vi "CountTeeth.vi"(8 "Falling Threshold":dbl, 9 "Rising Threshold":dbl, 10 "Direction":bool, 11 "Array":dbl[](array[numeric])) -> (0 "Gear Count":i32)   [LabVIEW 2017]
uses:
  ToothState.ctl
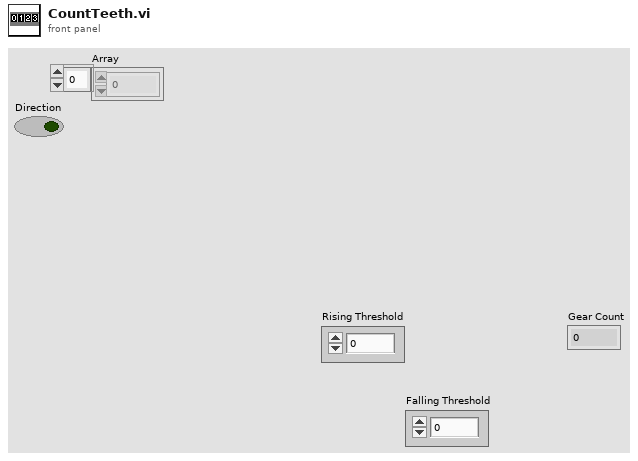
[diagram p1: front panel]
types:
  T1 = typedef "ToothState.ctl" = enum16{"Initialize State", "Rising ", "Falling"}
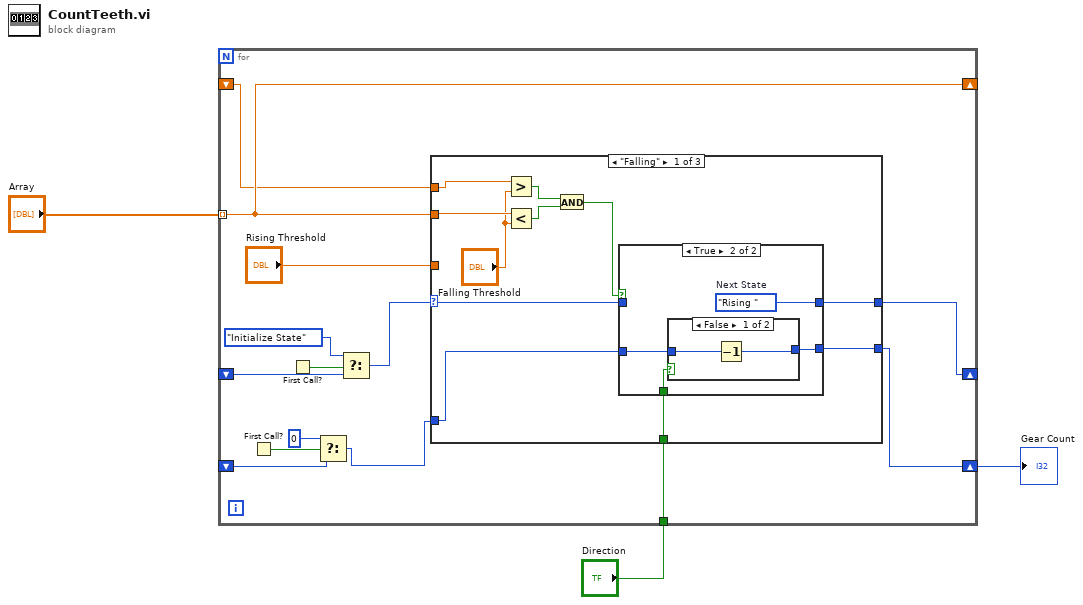
[diagram p0: block diagram]
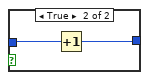
[diagram p3: hidden frame]
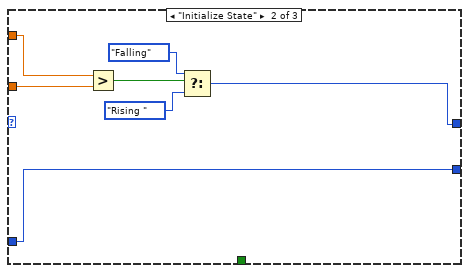
[diagram p4: hidden frame]
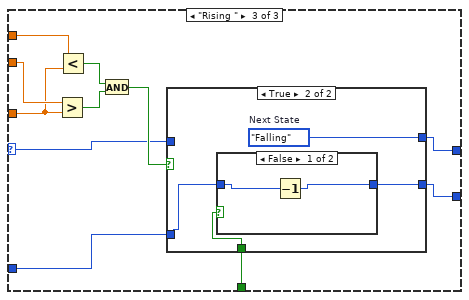
[diagram p5: hidden frame]
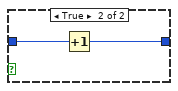
[diagram p7: hidden frame]
diagram:
  n1 = for {
    tunnel: "Array" -> [w17] mode=indexing
    shift-right: [w17] -> _
    shift-left: _ -> [w16]
    shift-right: [w15] -> _
    shift-left: _ -> [w11]
    shift-right: [w6] -> w3
    shift-left: _ -> [w7]
    tunnel: "Direction" -> [w5]
    n2 = First Call?() -> (First Call?: T/F=w9:bool)
    n3 = First Call?() -> (First Call?: T/F=w13:bool)
    n4 = Select(t=0, s=w9, f=w7) -> (s? t:f=w8:i32)
    n5 = Select(t=ToothState."Initialize State" ("Enum"), s=w13, f=w11) -> (s? t:f=w10:T1)
    n6 = case shown="\"Falling\"" w10 {
      selector: w10 -> [w19 _ w47]
      tunnel: w17 -> [w28 w45 w56]
      tunnel: w16 -> [w27 _ w55]
      tunnel: [w22 w40 w48] -> w15
      tunnel: w8 -> [w21 w39 w50]
      tunnel: [w20 w39 w49] -> w6
      tunnel: "Rising Threshold" -> [_ w44 w54]
      tunnel: w5 -> [w18 _ w46]
      frame "Falling" {
        n7 = Greater?(x=w27, y="Falling Threshold") -> (0:w25:bool)
        n8 = Less?(x=w28, y="Falling Threshold") -> (x < y?=w24:bool)
        n9 = And(x=w25, y=w24) -> (x .and. y?=w23:bool)
        n10 = case shown="True" w23 {
          tunnel: [w29 w34] -> w22
          tunnel: w21 -> [w30 w33]
          tunnel: [w30 w32] -> w20
          tunnel: w19 -> [w29 _]
          tunnel: w18 -> [_ w31]
          frame False {
          }
          frame True {
            w34 = ToothState."Rising "  # Next State
            n11 = case shown="False" w31 {
              tunnel: w33 -> [w36 w38]
              tunnel: [w35 w37] -> w32
              frame False {
                n12 = Decrement(x=w36) -> (x-1=w35:i32)
              }
              frame True {
                n13 = Increment(x=w38) -> (x+1=w37:i32)
              }
            }
          }
        }
      }
      frame "Initialize State" {
        n14 = Greater?(x=w45, y=w44) -> (0:w43:bool)
        n15 = Select(t=ToothState."Falling" ("Enum"), s=w43, f=ToothState."Rising " ("Enum")) -> (s? t:f=w40:T1)
      }
      frame "Rising " {
        n16 = Greater?(x=w56, y=w54) -> (0:w53:bool)
        n17 = Less?(x=w55, y=w54) -> (x < y?=w52:bool)
        n18 = And(x=w52, y=w53) -> (x .and. y?=w51:bool)
        n19 = case shown="True" w51 {
          tunnel: w50 -> [w58 w62]
          tunnel: [w58 w61] -> w49
          tunnel: [w57 w60] -> w48
          tunnel: w47 -> [w57 _]
          tunnel: w46 -> [_ w59]
          frame False {
          }
          frame True {
            w60 = ToothState."Falling"  # Next State
            n20 = case shown="False" w59 {
              tunnel: w62 -> [w64 w66]
              tunnel: [w63 w65] -> w61
              frame False {
                n21 = Decrement(x=w64) -> (x-1=w63:i32)
              }
              frame True {
                n22 = Increment(x=w66) -> (x+1=w65:i32)
              }
            }
          }
        }
      }
    }
  }
  "Gear Count" <- w3
